vi "Write RunVirtual.vi"(8 "error in (no error)":errorcluster, 10 "RunVirtual?":bool, 11 "Driver in":refnum<class "Driver.lvclass">) -> (0 "error out":errorcluster, 3 "Driver out":refnum<class "Driver.lvclass">)   [LabVIEW 2013, in "Driver.lvlib" / "Driver.lvclass"]
uses:
  Driver.lvclass
  Driver.lvclass/Driver.ctl
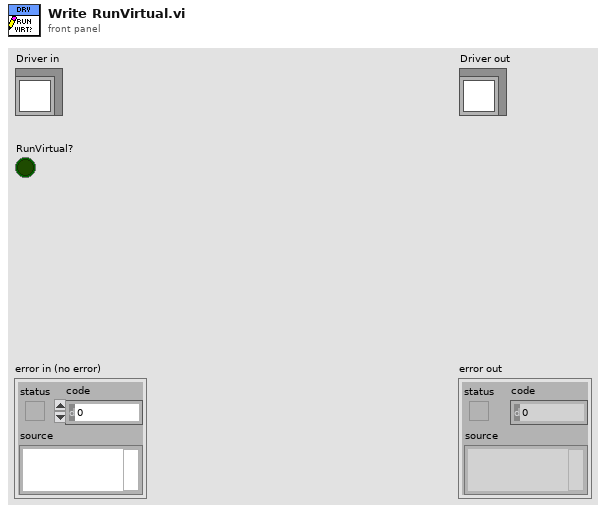
[diagram p1: front panel]
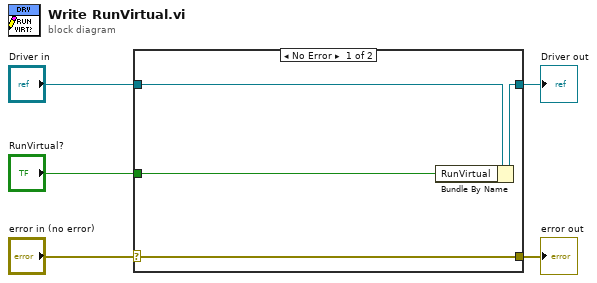
[diagram p0: block diagram]
diagram:
  n1 = case shown="No Error" "error in (no error)" {
    selector: "error in (no error)" -> [w9 w10]
    tunnel: [w9 w10] -> w4
    tunnel: [w7 w11] -> w2
    tunnel: "Driver in" -> [w8 w11]
    tunnel: "RunVirtual?" -> [w6 _]
    frame No Error {
      n2 = Bundle By Name(cluster=w8, "RunVirtual"=w6) -> (w7:refnum<class "Driver.lvclass">)
    }
    frame Error {
    }
  }
  "error out" <- w4
  "Driver out" <- w2
